vi "Get Item Names.vi"(8 "error in (no error)":errorcluster, 11 "Assembly Run in":refnum<class "Assembly Run.lvclass">) -> (0 "error out":errorcluster, 2 "Item names":string[][](array[string]), 3 "Assembly Run out":refnum<class "Assembly Run.lvclass">)   [LabVIEW 2019, in "Assembly Run.lvclass"]
uses:
  Assembly Run.lvclass
  Assembly Run.lvclass/Assembly Run.ctl
  Routine/Routine.lvclass
  Workspace/Fixture.lvclass
panel:
  out "transposed array":string[][](array[string])
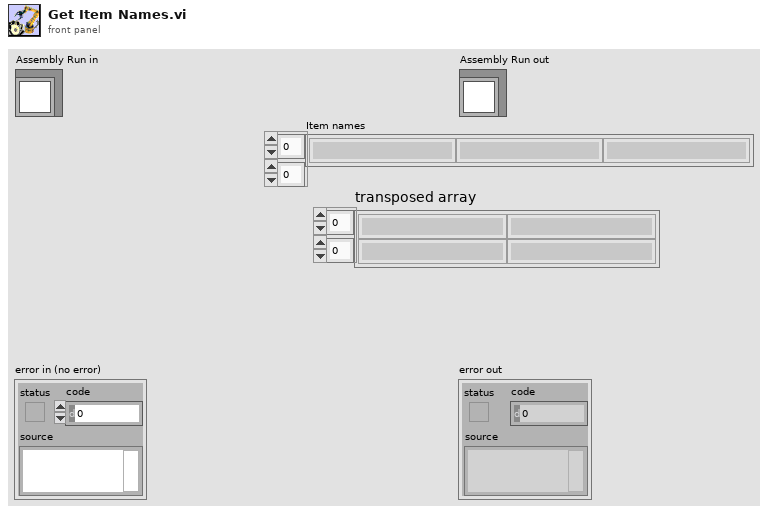
[diagram p1: front panel]
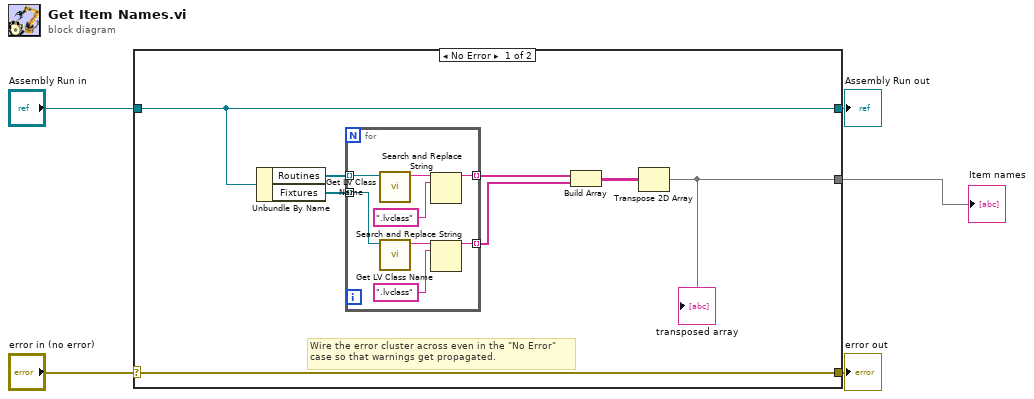
[diagram p0: block diagram]
diagram:
  n1 = case shown="No Error" "error in (no error)" {
    selector: "error in (no error)" -> [w13 w23]
    tunnel: [w13 w23] -> w4
    tunnel: [w6 w22] -> w2
    tunnel: "Assembly Run in" -> [w6 w22]
    tunnel: [w9 _] -> w1
    frame No Error {
      # "Wire the error cluster across even in the \"No Error\"\ncase so that warnings get propagated."
      n2 = Unbundle By Name(w6) -> ("Routines"=w11:refnum<class "Routine.lvclass">[], "Fixtures"=w12:refnum<class "Fixture.lvclass">[])
      n3 = for {
        tunnel: w11 -> [w21] mode=indexing
        tunnel: [w18] -> w8 mode=indexing
        tunnel: w12 -> [w17] mode=indexing
        tunnel: [w14] -> w7 mode=indexing
        n4 = call <vilib>:"Get LV Class Name.vi"("object"=w21) -> ("class name"=w19:string)  [unwired: 9 in, 1 out]
        n5 = call <vilib>:"Get LV Class Name.vi"("object"=w17) -> ("class name"=w16:string)  [unwired: 9 in, 1 out]
        n6 = Search and Replace String(input string=w19, search string=".lvclass" ("substring (\"\")")) -> (result string=w18:string)  [unwired: 6 in, 3 out]
        n7 = Search and Replace String(input string=w16, search string=".lvclass" ("substring (\"\")")) -> (result string=w14:string)  [unwired: 6 in, 3 out]
      }
      n8 = Build Array(w8, w7) -> (w10:string[][])
      n9 = Transpose 2D Array(2D array=w10) -> (transposed array=w9:string[][])
      "transposed array" <- w9
    }
    frame Error {
    }
  }
  "error out" <- w4
  "Assembly Run out" <- w2
  "Item names" <- w1
